vi "samplePlaybackTest.vi"() -> ()   [LabVIEW 2009]
uses:
  Debug/samplePlaybackGenerator.dll
panel:
  out "pOutput":dbl[](array[numeric])
  in  "dimension size":i32
  in  "tStep":dbl
  in  "t0":dbl
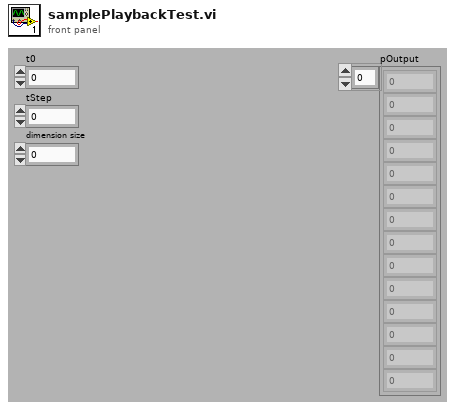
[diagram p1: front panel]
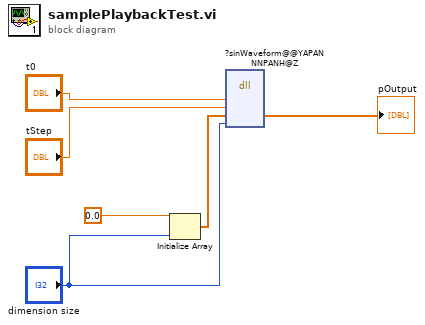
[diagram p0: block diagram]
diagram:
  n1 = Initialize Array(0.0 ("element"), "dimension size") -> (w3:dbl[])
  n2 = dll-call lib="C:/Documents and Settings/sauna/My Documents/Visual Studio 2008/Projects/samplePlaybackGenerator/Debug/samplePlaybackGenerator.dll" fn="?sinWaveform@@YAPANNNPANH@Z"("t0"="t0", "tStep"="tStep", "pOutput"=w3, "outputLength"="dimension size") -> ("pOutput"=→"pOutput":dbl[])  [unwired: 7 in, 2 out]
